vi "Get Variant Message.vi"(8 "error in (no error)":errorcluster, 11 "Message Boolean in":refnum<class "Message Boolean.lvclass">) -> (0 "error out":errorcluster, 1 "Value":variant, 2 "Name":string, 3 "Message Boolean out":refnum<class "Message Boolean.lvclass">)   [LabVIEW 2016, in "Stream Mediator.lvlib" / "Message Boolean.lvclass"]
doc: "--\nCopyright © 2017 Composed SystemsI All rights reserved.\n\nAuthor: Jon McBee <jon.mcbee@composed.io>\n\nThis library is provided \"AS IS\" ,WITHOUT WARRANTIES OR\nCONDITIONS OF ANY KIND, either express or implied.\n\nComposed Systems -- composed.io\n\nStream 0.0.1.1\nJon McBee - Composed Systems\nCopyright (c) 2017, Composed Systems"
uses:
  <userlib>/Composed Systems/Stream/Mediator/Classes/Message Boolean/Message Boolean.lvclass
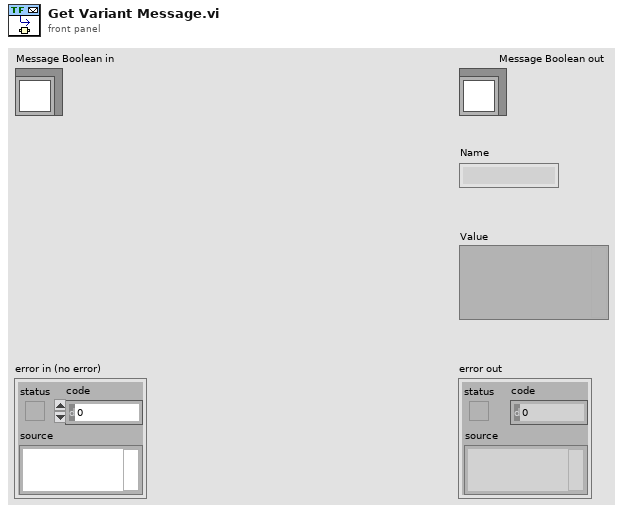
[diagram p1: front panel]
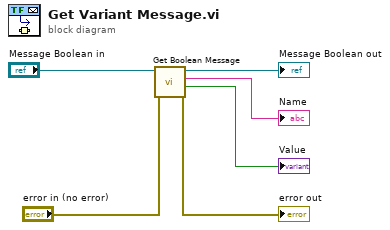
[diagram p0: block diagram]
diagram:
  n1 = call <userlib>:"Get Boolean Message.vi"("error in (no error)"="error in (no error)", "Message Boolean in"="Message Boolean in") -> ("error out"=→"error out":errorcluster, "Value"=→"Value":bool, "Name"=→"Name":string, "Message Boolean out"=→"Message Boolean out":refnum<class "Message Boolean.lvclass">)  [unwired: 6 in]
